vi "set controllers.vi"() -> ()   [LabVIEW 2018]
panel:
  out "Controller ID# Found":u8
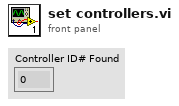
[diagram p1: front panel]
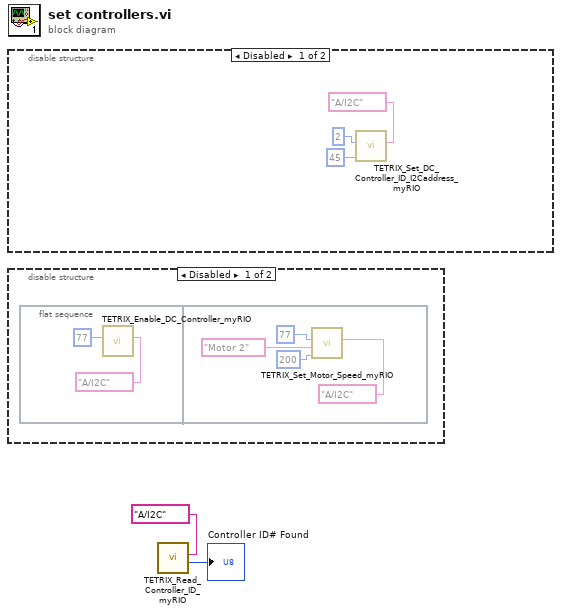
[diagram p0: block diagram]
diagram:
  n1 = disable-structure shown="Disabled" {
    frame Disabled {
      n2 = call <vilib>:"TETRIX_Set_DC_Controller_ID_I2Caddress_myRIO.vi"("myRIO MXP Port A/B"=tag "A/I2C", "New ID# / I2C Address"=u8 45, "Current ID#  / I2C Address"=u8 2) -> ()  [unwired: 4 in, 1 out]
    }
    frame Enabled {
    }
  }
  n3 = disable-structure shown="Disabled" {
    frame Disabled {
      n4 = flat-sequence {
        frame #0 {
          n5 = call <vilib>:"TETRIX_Enable_DC_Controller_myRIO.vi"("myRIO MXP Port A/B"=tag "A/I2C", "Controller ID#  (I2C Address)"=u8 77) -> ()  [unwired: 5 in, 1 out]
        }
        frame #1 {
          n6 = call <vilib>:"TETRIX_Set_Motor_Speed_myRIO.vi"("myRIO MXP Port A/B"=tag "A/I2C", "Constant Speed (Degrees per second). Sign (+/-)  sets direction."=i16 200, "Select Channel"="Motor 2", "Controller ID#  (I2C Address)"=u8 77) -> ()  [unwired: 3 in, 1 out]
        }
      }
    }
    frame Enabled {
    }
  }
  n7 = call <vilib>:"TETRIX_Read_Controller_ID_myRIO.vi"("myRIO MXP Port A/B"=tag "A/I2C") -> ("Controller ID# Found"=→"Controller ID# Found":u8)  [unwired: 5 in, 1 out]
